vi "6_Filtering.vi"() -> ()   [LabVIEW 2015]
uses:
  C:/Users/MX-Microscope/Documents/LabVIEW Data/lvoop_campus_2018/Detector_Class/Swabian/time_tagger_vis/TTCSharp32.dll
  TTCSharp32.dll
panel:
  out "Test signal only on channel 7":dbl[](array[numeric])
  out "Test signal on channel 0 and 7":dbl[](array[numeric])
  # "counts / s"
  # "channel 0"
  # "counts / s"
  # "channel 7 (filtered)"
  # "channel 0"
  # "counts / s"
  # "channel 7 (filtered)"
  # "counts / s"
  # "Here, we have used the event filter between channel 0 and\nchannel 7 to suppress time tags on channel 7. The filter drops time tags on\nchannel 7 unless they were preceded by a tag on channel 0. First, since the tags are\nsimultaneous on both channels, but there is a finite jitter the count rate on channel 7\nis reduced by some amount. Now, as we disable the test signal on channel 0, all time\ntags on channel 7 are suppressed and a count rate of 0 is measured, even though the test\nsignal is active. The filtering is useful to tame signals with data rates > 8 MHz such as\nsynchronization signals from pulsed lasers in fluorescence lifetime measurements."
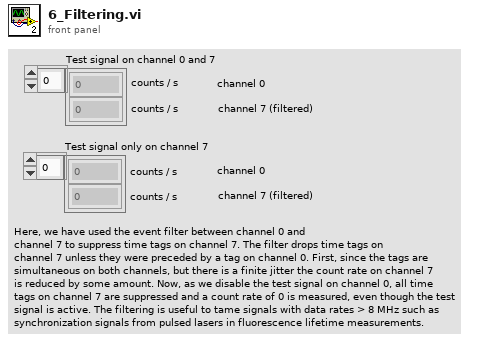
[diagram p1: front panel]
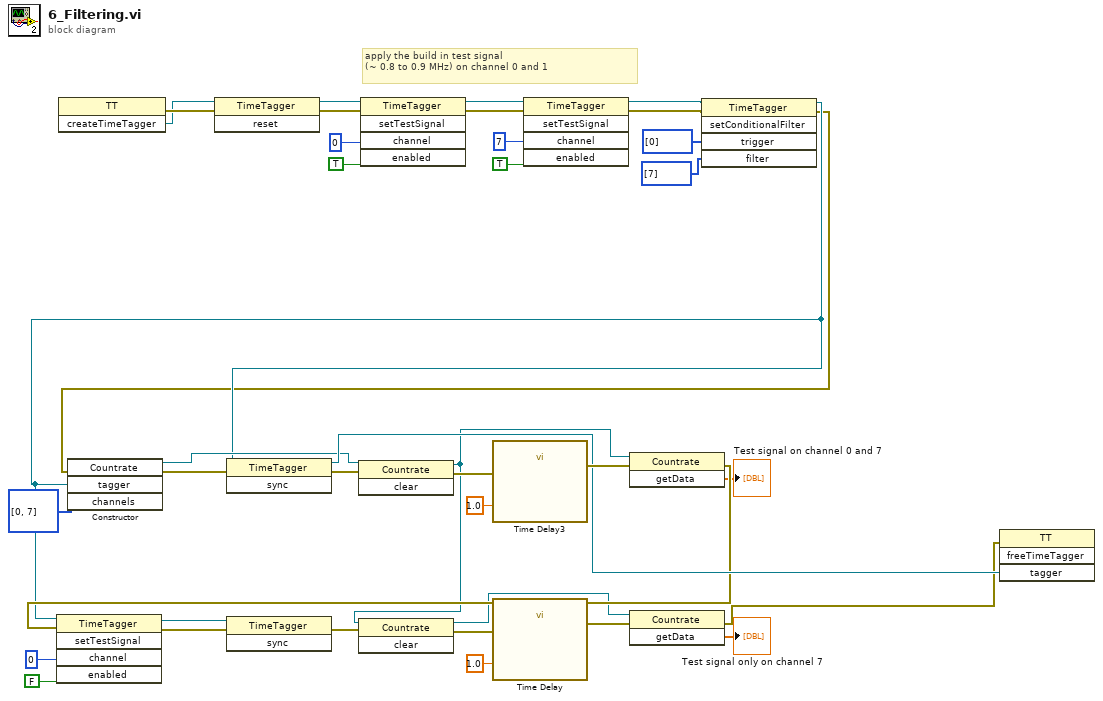
[diagram p0: block diagram]
diagram:
  # "apply the build in test signal\n(~ 0.8 to 0.9 MHz) on channel 0 and 1"
  n1 = invoke class="TT" method="createTimeTagger"() -> (error out=w34:errorcluster, "createTimeTagger"=w33:refnum<k24>)  [unwired: 3 in, 1 out]
  n2 = invoke class="TimeTagger" method="reset"(reference=w33, error in=w34) -> (reference out=w29:refnum<k24>, error out=w30:errorcluster)  [unwired: 1 in, 1 out]
  n3 = invoke class="TimeTagger" method="setTestSignal"(reference=w29, error in=w30, "channel"=u32 0, "enabled"=TRUE) -> (reference out=w31:refnum<k24>, error out=w32:errorcluster)  [unwired: 1 in, 3 out]
  n4 = invoke class="TimeTagger" method="setTestSignal"(reference=w31, error in=w32, "channel"=u32 7, "enabled"=TRUE) -> (reference out=w4:refnum<k24>, error out=w3:errorcluster)  [unwired: 1 in, 3 out]
  n5 = invoke class="TimeTagger" method="setConditionalFilter"(reference=w4, error in=w3, "trigger"=u32[] [0], "filter"=u32[] [7]) -> (reference out=w2:refnum<k24>, error out=w1:errorcluster)  [unwired: 1 in, 3 out]
  n6 = constructor class="Countrate"(error in=w1, "tagger"=w2, "channels"=u32[] [0, 7]) -> (reference out=w10:refnum<k24>, error out=w23:errorcluster)  [unwired: 2 in, 3 out]
  n7 = invoke class="TimeTagger" method="sync"(reference=w2, error in=w23) -> (reference out=w24:refnum<k24>, error out=w25:errorcluster)  [unwired: 1 in, 1 out]
  n8 = invoke class="Countrate" method="clear"(reference=w10, error in=w25) -> (reference out=w9:refnum<k24>, error out=w28:errorcluster)  [unwired: 1 in, 1 out]
  n9 = call "Time Delay3"("error in (no error)"=w28, "Delay Time (s)"=1.0) -> ("error out"=w26:errorcluster)  [unwired: 9 in]
  n10 = invoke class="Countrate" method="getData"(reference=w9, error in=w26) -> (error out=w19:errorcluster, "getData"=→"Test signal on channel 0 and 7":dbl[])  [unwired: 1 in, 1 out]
  n11 = invoke class="TimeTagger" method="setTestSignal"(reference=w2, error in=w19, "channel"=u32 0, "enabled"=FALSE) -> (reference out=w12:refnum<k24>, error out=w11:errorcluster)  [unwired: 1 in, 3 out]
  n12 = invoke class="TimeTagger" method="sync"(reference=w12, error in=w11) -> (error out=w14:errorcluster)  [unwired: 1 in, 2 out]
  n13 = invoke class="Countrate" method="clear"(reference=w9, error in=w14) -> (reference out=w8:refnum<k24>, error out=w17:errorcluster)  [unwired: 1 in, 1 out]
  n14 = call "Time Delay"("error in (no error)"=w17, "Delay Time (s)"=1.0) -> ("error out"=w15:errorcluster)  [unwired: 9 in]
  n15 = invoke class="Countrate" method="getData"(reference=w8, error in=w15) -> (error out=w7:errorcluster, "getData"=→"Test signal only on channel 7":dbl[])  [unwired: 1 in, 1 out]
  n16 = invoke class="TT" method="freeTimeTagger"(error in=w7, "tagger"=w24) -> ()  [unwired: 2 in, 4 out]
